vi "ellipseConversion.vi"(6 "XY ellipse 2":cluster{"x":dbl[], "y":dbl[]}) -> (5 "Array":cluster{dbl, dbl}[](array[cluster]))   [LabVIEW 2014]
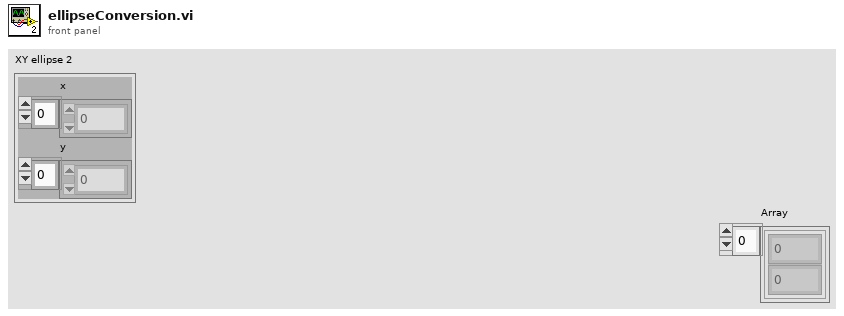
[diagram p1: front panel]
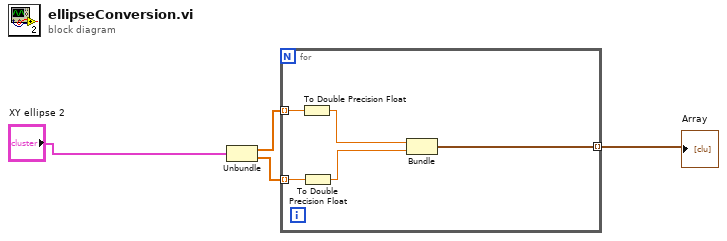
[diagram p0: block diagram]
diagram:
  n1 = Unbundle("XY ellipse 2") -> ("x"=w4:dbl[], "y"=w1:dbl[])
  n2 = for {
    tunnel: w4 -> [w9] mode=indexing
    tunnel: w1 -> [w8] mode=indexing
    tunnel: [w5] -> w3 mode=indexing
    n3 = To Double Precision Float(number=w9) -> (double precision float=w7:dbl)
    n4 = To Double Precision Float(number=w8) -> (double precision float=w6:dbl)
    n5 = Bundle(w7, w6) -> (w5:cluster{dbl, dbl})  [unwired: 1 in]
  }
  "Array" <- w3
